vi "fgv_PXI-5110_config.vi"(7 "cmd":T2, 11 "cfg":T1={"visa"="Dev1", "Channel Name"="0", "Enforce Realtime"=TRUE, "Vertical Range"=5.0, "Min Sample Rate"=10000000.0, "Min Record Length"=1000, "Actual Record Length"=1000, "Actual Sample Rate"=10000000.0, "Timeout (s)"=5.0, "Vertical Offset"=0.0, "Probe Attenuation"=1.0, "Input Impedance"=0, "Maximum Input Frequency"=0.0, "Vertical Coupling"=1, "Trigger"={"Coupling"=1, "Trigger Slope"=0, "Trigger Level"=0.0, "Trigger Source"="0", "Trigger Delay"=0.0, "Reference Position"=50.0, "Trigger Modifier"=2, "Auto Triggered"=FALSE}} {"Trigger"."Trigger Modifier" items=["None"=1, "Auto Trigger"=2]; "Trigger"."Reference Position" format="%.1f"; "Trigger"."Trigger Delay" format="%#.4p"; "Trigger"."Trigger Level" format="%.2f"; "Trigger"."Trigger Slope" items=["Positive", "Negative"]; "Trigger"."Coupling" items=["AC"=0, "DC"=1, "HF Reject"=3, "LF Reject"=4, "AC Plus HF Reject"=1001]; "Vertical Coupling" items=["AC", "DC", "Ground"]; "Maximum Input Frequency" format="%.2f"; "Input Impedance" items=["1 mega ohm"=0, "50 ohms"=2]; "Probe Attenuation" format="%.1f"; "Vertical Offset" format="%.2p"; "Timeout (s)" format="%.2f"; "Actual Sample Rate" format="%#.2p"; "Min Sample Rate" step=1000000.0 format="%#.2p"; "Vertical Range" format="%.2f"}) -> (3 "cfg 2":T1={"visa"="Dev1", "Channel Name"="0", "Enforce Realtime"=TRUE, "Vertical Range"=5.0, "Min Sample Rate"=10000000.0, "Min Record Length"=1000, "Actual Record Length"=1000, "Actual Sample Rate"=10000000.0, "Timeout (s)"=5.0, "Vertical Offset"=0.0, "Probe Attenuation"=1.0, "Input Impedance"=0, "Maximum Input Frequency"=0.0, "Vertical Coupling"=1, "Trigger"={"Coupling"=1, "Trigger Slope"=0, "Trigger Level"=0.0, "Trigger Source"="0", "Trigger Delay"=0.0, "Reference Position"=50.0, "Trigger Modifier"=2, "Auto Triggered"=FALSE}} {"Trigger"."Trigger Modifier" items=["None"=1, "Auto Trigger"=2]; "Trigger"."Reference Position" format="%.1f"; "Trigger"."Trigger Delay" format="%#.4p"; "Trigger"."Trigger Level" format="%.2f"; "Trigger"."Trigger Slope" items=["Positive", "Negative"]; "Trigger"."Coupling" items=["AC"=0, "DC"=1, "HF Reject"=3, "LF Reject"=4, "AC Plus HF Reject"=1001]; "Vertical Coupling" items=["AC", "DC", "Ground"]; "Maximum Input Frequency" format="%.2f"; "Input Impedance" items=["1 mega ohm"=0, "50 ohms"=2]; "Probe Attenuation" format="%.1f"; "Vertical Offset" format="%.2p"; "Timeout (s)" format="%.2f"; "Actual Sample Rate" format="%#.2p"; "Min Sample Rate" step=1000000.0 format="%#.2p"; "Vertical Range" format="%.2f"})   [LabVIEW 2021]
uses:
  ctrl/ini-rw.ctl
  ctrl/5110_trigger.ctl
panel:
  # "Vertical"
  # "Channel"
  # "Horizontal"
  # "Vertical"
  # "Channel"
  # "Horizontal"
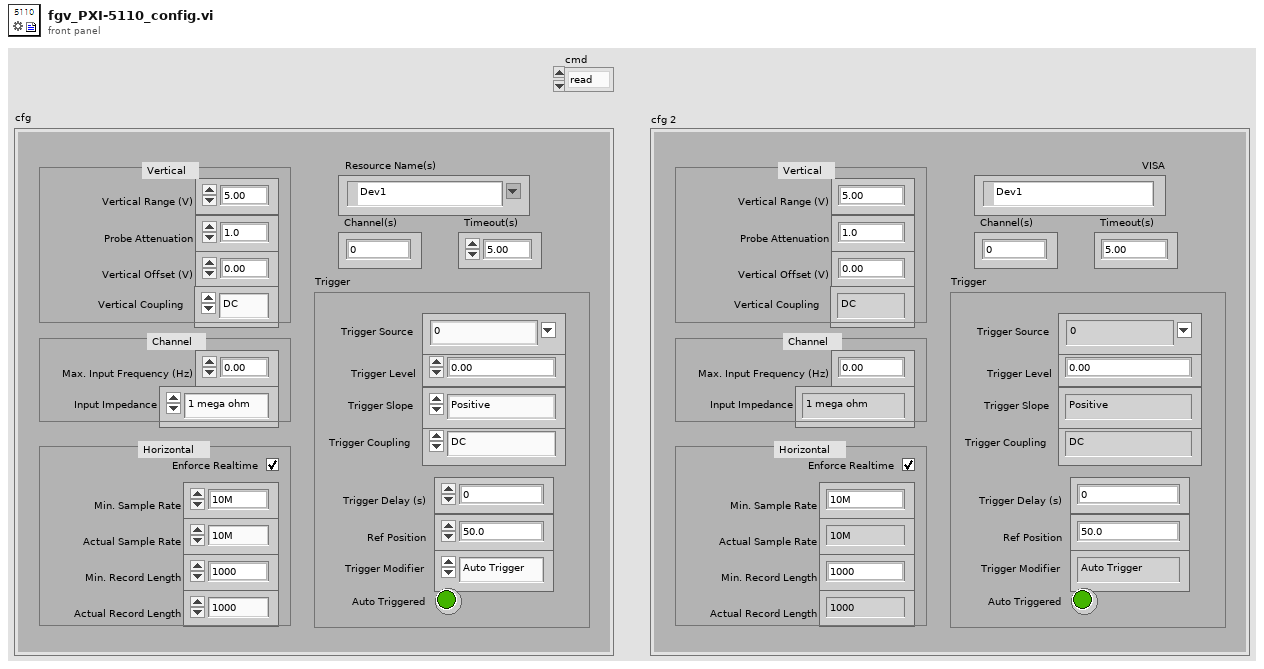
[diagram p1: front panel]
types:
  T1 = typedef "5110_trigger.ctl" = cluster{"visa":refnum<k15>, "Channel Name":string, "Enforce Realtime":bool, "Vertical Range":dbl, "Min Sample Rate":dbl, "Min Record Length":i32, "Actual Record Length":i32, "Actual Sample Rate":dbl, "Timeout (s)":dbl, "Vertical Offset":dbl, "Probe Attenuation":dbl, "Input Impedance":u32, "Maximum Input Frequency":dbl, "Vertical Coupling":i32, "Trigger":cluster{"Coupling":u16, "Trigger Slope":i32, "Trigger Level":dbl, "Trigger Source":string, "Trigger Delay":dbl, "Reference Position":dbl, "Trigger Modifier":i32, "Auto Triggered":bool}}
  T2 = typedef "ini-rw.ctl" = enum16{"read", "write", "ini"}
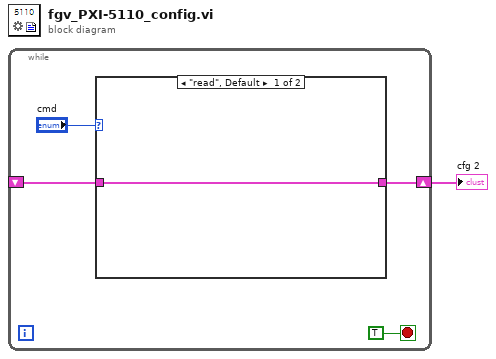
[diagram p0: block diagram]
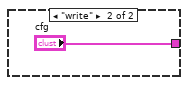
[diagram p2: hidden frame]
diagram:
  n1 = while {
    shift-right: [w3] -> w1
    shift-left: _ -> [w2]
    stop <- TRUE stop-if-true
    n2 = case shown="\"read\", Default" "cmd" {
      tunnel: [w6 "cfg"] -> w3
      tunnel: w2 -> [w6 _]
      frame "read", Default {
      }
      frame "write" {
      }
    }
  }
  "cfg 2" <- w1
